vi "visualisation_&_control.vi"(11 "motor speeds":cluster{"M1":dbl, "M2":dbl} {"M2" scale=0.0..255.0; "M1" scale=0.0..255.0}) -> ()   [LabVIEW 2022 SP3]
uses:
  <vilib>/addons/control/pid/pid.llb/PID (DBL).vi
  <vilib>/addons/control/pid/NI_PID_pid.lvlib
panel:
  in  "rounded":bool
  in  "Motors OFF":bool
  in  "PID":bool
  in  "PID Gains":cluster{"Kp":ext, "Ki":ext, "Kd":ext}={"Kp"=0.2, "Ki"=0.0, "Kd"=0.0007}
  in  "stop code":bool
  out "Target Roll":dbl
  out "Measured Roll":dbl
  in  "target slider":dbl(slide) scale=-20.0..20.0
  out "Waveform Chart":dynamicdata(graph)
  in  "port":u16=8000
  in  "address":string="192.168.137.100"
  # "Motors ON"
  # "Manual"
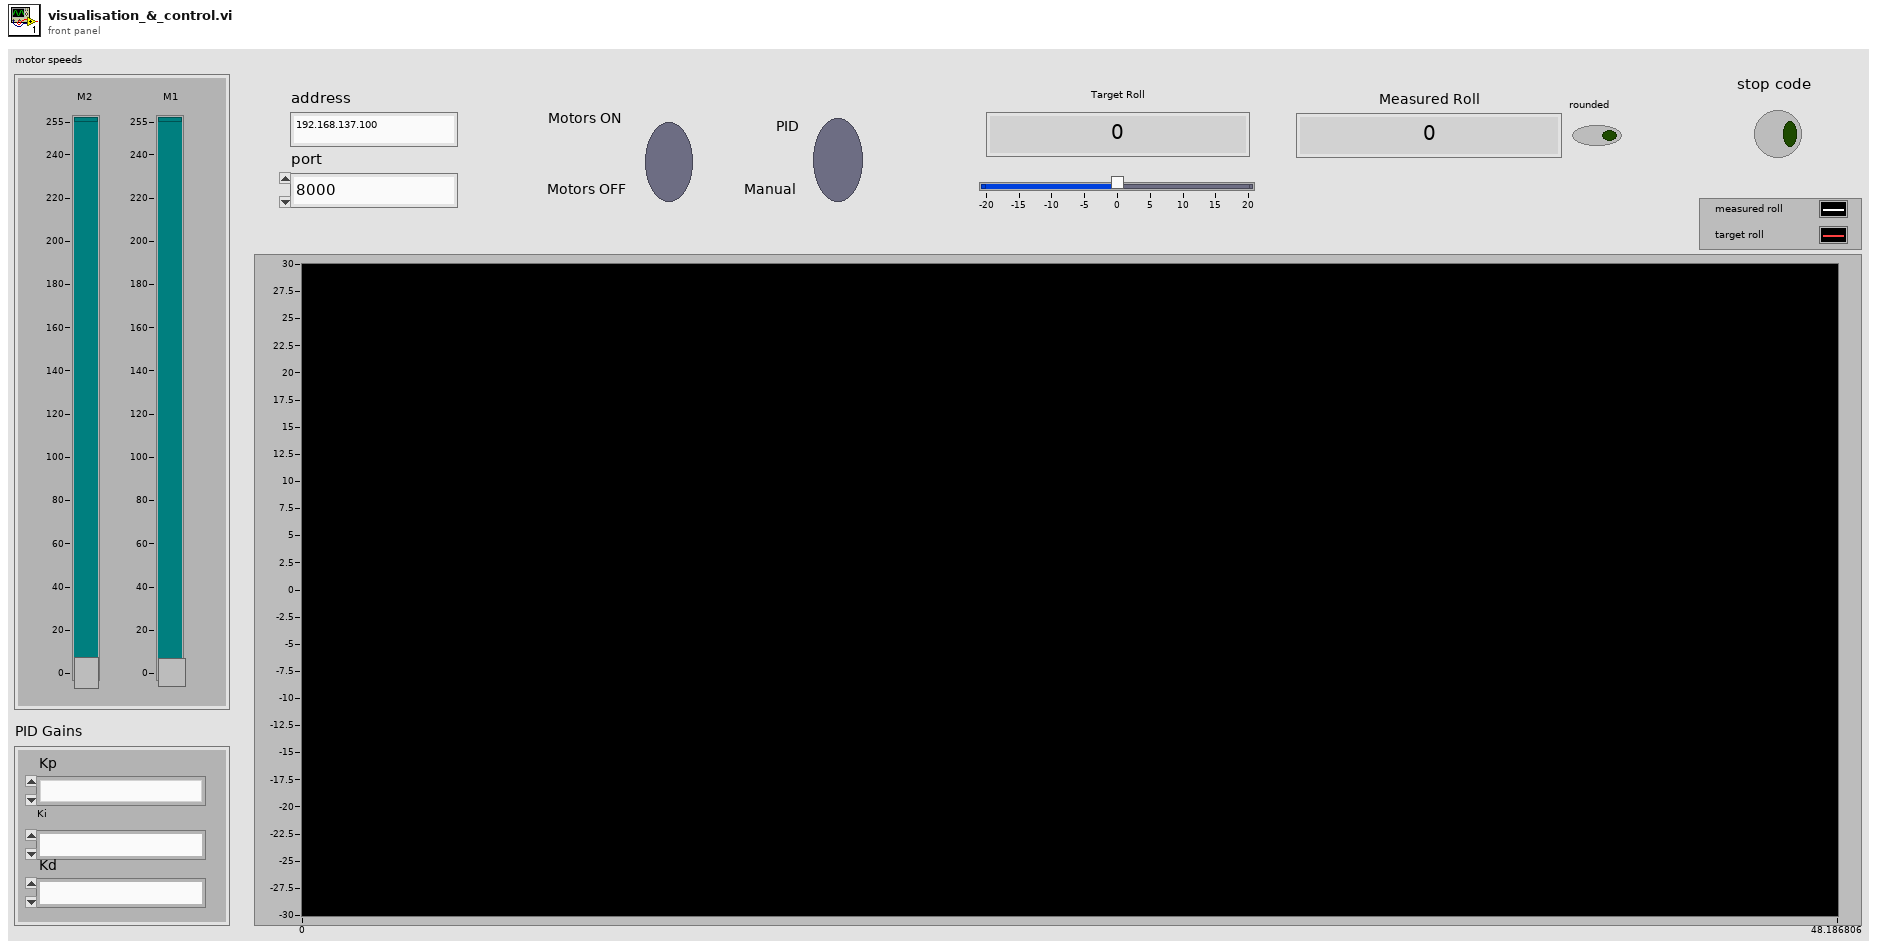
[diagram p1: front panel]
types:
  T1 = enum16{"Standard", "Buffered", "CRLF", "Immediate"}
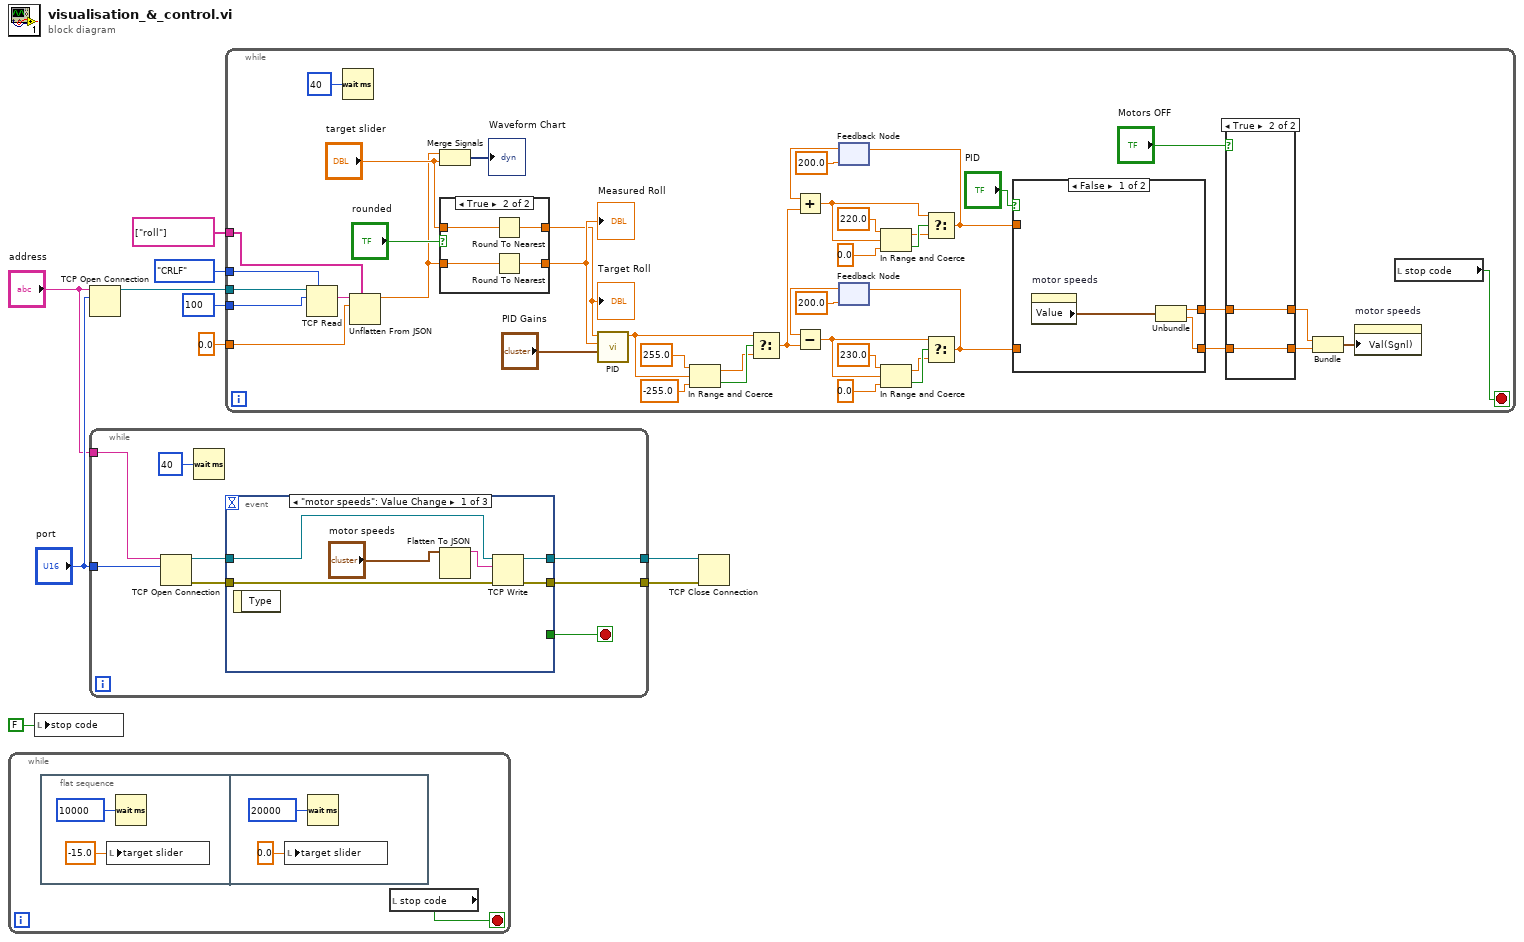
[diagram p0: block diagram]
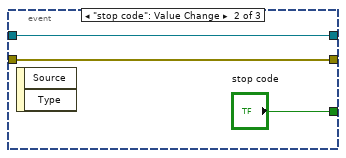
[diagram p2: hidden frame]
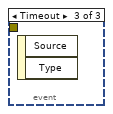
[diagram p3: hidden frame]
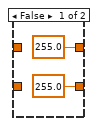
[diagram p5: hidden frame]
diagram:
  n1 = while {
    stop <- w11 stop-if-true
    n2 = flat-sequence {
      frame #0 {
        n3 = local write "target slider"(-15.0 ("target slider")) -> ()
        n4 = Wait (ms)(milliseconds to wait=u32 10000) -> ()  [unwired: 1 out]
      }
      frame #1 {
        n5 = local write "target slider"(0.0 ("target slider")) -> ()
        n6 = Wait (ms)(milliseconds to wait=u32 20000) -> ()  [unwired: 1 out]
      }
    }
    n7 = local read "stop code"() -> (w11:bool)
  }
  n8 = local write "stop code"(FALSE ("stop code")) -> ()
  n9 = TCP Open Connection(address="address", remote port or service name="port") -> (connection ID=w6:refnum<k5>)  [unwired: 3 in, 1 out]
  n10 = while {
    tunnel: "port" -> [w23]
    tunnel: "address" -> [w22]
    tunnel: [w17] -> w2
    tunnel: [w16] -> w1
    stop <- w18 stop-if-true
    n11 = TCP Open Connection(address=w22, remote port or service name=w23) -> (connection ID=w20:refnum<k5>, error out=w21:errorcluster)  [unwired: 3 in]
    n12 = Wait (ms)(milliseconds to wait=u32 40) -> ()  [unwired: 1 out]
    n13 = event shown="[0] \"motor speeds\": Value Change" {
      selector: _ -> [_ _ _]
      dyn-events: _ -> [_ _ _]
      timeout: _ -> [_ _ _]
      tunnel: w21 -> [w28 w31 _]
      tunnel: w20 -> [w26 w32 _]
      tunnel: [w25 w31 _] -> w17
      tunnel: [w24 w32 _] -> w16
      tunnel: [_ "stop code" _] -> w18
      event "motor speeds": Value Change {
        n14 = event-data() -> ()  [unwired: 1 in, 1 out]
        n15 = Flatten To JSON(anything="motor speeds") -> (JSON string=w27:string)  [unwired: 2 in, 1 out]
        n16 = TCP Write(connection ID=w26, data in=w27, error in (no error)=w28) -> (connection ID out=w24:refnum<k5>, error out=w25:errorcluster)  [unwired: 1 in, 1 out]
      }
      event "stop code": Value Change {
        n17 = event-data() -> ()  [unwired: 1 in, 2 out]
      }
      event Timeout {
        n18 = event-data() -> ()  [unwired: 1 in, 2 out]
      }
    }
  }
  n19 = while {
    tunnel: 100 ("bytes to read") -> [w75]
    tunnel: T1."CRLF" ("mode (standard)") -> [w74]
    tunnel: string[] ["roll"] ("path") -> [w72]
    tunnel: 0.0 -> [w71]
    tunnel: w6 -> [w70]
    stop <- w38 stop-if-true
    n20 = TCP Read(connection ID=w70, bytes to read=w75, 7:w74) -> (data out=w76:string)  [unwired: 2 in, 2 out]
    n21 = Wait (ms)(milliseconds to wait=u32 40) -> ()  [unwired: 1 out]
    n22 = Unflatten From JSON(path=w72, JSON string=w76, type and defaults=w71) -> (value=w35:dbl)  [unwired: 4 in, 1 out]
    n23 = Merge Signals(w35, "target slider") -> (→"Waveform Chart":dynamicdata)
    n24 = case shown="True" "rounded" {
      tunnel: "target slider" -> [w78 w82]
      tunnel: [w78 w81] -> w33
      tunnel: w35 -> [w77 w80]
      tunnel: [w77 w79] -> w34
      frame False {
      }
      frame True {
        n25 = Round To Nearest(number=w82) -> (nearest integer value=w81:dbl)
        n26 = Round To Nearest(number=w80) -> (nearest integer value=w79:dbl)
      }
    }
    "Measured Roll" <- w34
    "Target Roll" <- w33
    n27 = call-poly <vilib>:"PID.vi"("PID gains"="PID Gains", "process variable"=w34, "setpoint"=w33) -> ("output"=w50:dbl)  [unwired: 7 in, 1 out]
    n28 = In Range and Coerce(upper limit=255.0, x=w50, lower limit=-255.0) -> (coerced(x)=w51:dbl, In Range?=w52:bool)
    n29 = Select(t=w50, s=w52, f=w51) -> (s? t:f=w49:dbl)
    n30 = feedback #1(200.0) -> (w67:dbl)
    n31 = Add(x=w67, y=w49) -> (x+y=w60:dbl)
    n32 = feedback #2(200.0) -> (w66:dbl)
    n33 = Subtract(x=w66, y=w49) -> (x-y=w54:dbl)
    n34 = In Range and Coerce(upper limit=220.0 ("y"), x=w60, lower limit=0.0 ("y")) -> (coerced(x)=w59:dbl, In Range?=w61:bool)
    n35 = In Range and Coerce(upper limit=230.0 ("y"), x=w54, lower limit=0.0 ("y")) -> (coerced(x)=w55:dbl, In Range?=w56:bool)
    n36 = Select(t=w60, s=w61, f=w59) -> (s? t:f=w45:dbl)
    n37 = feedback-in #1(w45) -> ()
    n38 = Select(t=w54, s=w56, f=w55) -> (s? t:f=w46:dbl)
    n39 = feedback-in #2(w46) -> ()
    n40 = case shown="False" "PID" {
      tunnel: w46 -> [_ w91]
      tunnel: [w87 w91] -> w44
      tunnel: [w88 w90] -> w42
      tunnel: w45 -> [_ w90]
      frame False {
        n41 = property on="motor speeds" class="Clust (strict)"() -> ("Value"=w89:cluster{"M1":dbl, "M2":dbl})  [unwired: 2 in, 2 out]
        n42 = Unbundle(w89) -> ("M1"=w88:dbl, "M2"=w87:dbl)
      }
      frame True {
      }
    }
    n43 = case shown="True" "Motors OFF" {
      tunnel: w44 -> [_ w86]
      tunnel: [255.0 ("y") w86] -> w43
      tunnel: w42 -> [_ w85]
      tunnel: [255.0 ("y") w85] -> w41
      frame False {
      }
      frame True {
      }
    }
    n44 = Bundle("y"=w41, "y"=w43) -> (w53:cluster{"y":dbl, "y":dbl})  [unwired: 1 in]
    n45 = property on="motor speeds" class="Clust (strict)"("Val(Sgnl)"=w53) -> ()  [unwired: 2 in, 2 out]
    n46 = local read "stop code"() -> (w38:bool)
  }
  n47 = TCP Close Connection(connection ID=w1, error in (no error)=w2) -> ()  [unwired: 1 in, 2 out]
